vi "VHM-getDataSetvi.vi"(8 "error in (no error)":errorcluster, 11 "VHM-VNA_Hardware_Manager in":refnum<class "VHM-VNA_Hardware_Manager.lvclass">) -> (0 "error out":errorcluster, 2 "VNA data":T2, 3 "VHM-VNA_Hardware_Manager out":refnum<class "VHM-VNA_Hardware_Manager.lvclass">)   [LabVIEW 2020, in "VHM-VNA_Hardware_Manager.lvlib" / "VHM-VNA_Hardware_Manager.lvclass"]
uses:
  VHM-VNA_Hardware_Manager.lvclass
  classes/vna-drivers/liteVNA/VD-VNA_data.ctl
  classes/vna-drivers/liteVNA/VD-data_read_status.ctl
  VHM-VNA_Hardware_Manager.lvclass/VHM-VNA_Hardware_Manager.ctl
  classes/vna-drivers/liteVNA/VD-LV-LiteVNA.lvclass
panel:
  out "Valid Data?":bool
  out "data status":T1
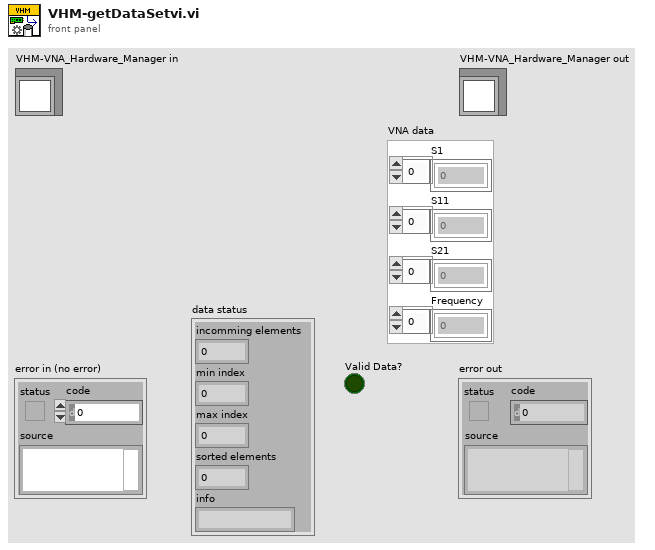
[diagram p1: front panel]
types:
  T1 = typedef "VD-LV-LiteVNA.lvclass/VD-data_read_status.ctl" = cluster{"incomming elements":i32, "min index":u16, "max index":u16, "sorted elements":i32, "info":string}
  T2 = typedef "VD-LV-LiteVNA.lvclass/VD-VNA_data.ctl" = cluster{"S1":cdb[], "S11":cdb[], "S21":cdb[], "Frequency":u64[]}
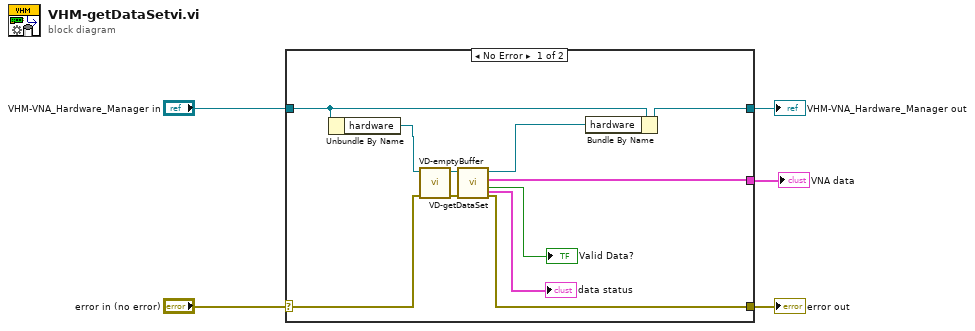
[diagram p0: block diagram]
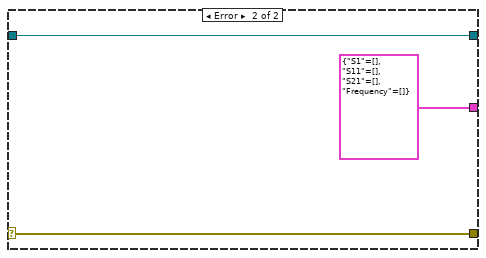
[diagram p2: hidden frame]
diagram:
  n1 = case shown="No Error" "error in (no error)" {
    selector: "error in (no error)" -> [w9 w19]
    tunnel: [w12 w19] -> w4
    tunnel: [w15 w18] -> w2
    tunnel: "VHM-VNA_Hardware_Manager in" -> [w16 w18]
    tunnel: [w13 T2 {"S1"=[], "S11"=[], "S21"=[], "Frequency"=[]} ("VNA data")] -> w1
    frame No Error {
      n2 = Unbundle By Name(w16) -> ("hardware"=w8:refnum<class "VD-LV-LiteVNA.lvclass">)
      n3 = call-dynamic "VD-emptyBuffer.vi"("error in (no error)"=w9, "VD-LV-LiteVNA in"=w8) -> ("error out"=w7:errorcluster, "VD-LV-LiteVNA out"=w6:refnum<class "VD-LV-LiteVNA.lvclass">)  [unwired: 5 in, 3 out]
      n4 = call-dynamic "VD-getDataSet.vi"("error in (no error)"=w7, "VD-LV-LiteVNA in"=w6) -> ("error out"=w12:errorcluster, "Valid Data?"=→"Valid Data?":bool, "VNA data"=w13:T2, "VD-LV-LiteVNA out"=w14:refnum<class "VD-LV-LiteVNA.lvclass">, "data status"=→"data status":T1)  [unwired: 5 in]
      n5 = Bundle By Name(cluster=w16, "hardware"=w14) -> (w15:refnum<class "VHM-VNA_Hardware_Manager.lvclass">)
    }
    frame Error {
    }
  }
  "error out" <- w4
  "VHM-VNA_Hardware_Manager out" <- w2
  "VNA data" <- w1
